vi "Do.vi"(8 "error in (no error)":errorcluster, 10 "Actor in":refnum<class "Actor.lvclass">, 11 "Configure Runt Trigger Source [RT] Msg":refnum<class "Configure Runt Trigger Source [RT] Msg.lvclass">) -> (0 "error out":errorcluster, 2 "Actor out":refnum<class "Actor.lvclass">)   [LabVIEW 2015, in "CS++Scope.lvlib" / "Configure Runt Trigger Source [RT] Msg.lvclass"]
doc: "This VI delivers the message to the actor by calling the appropriate method(s) on the actor."
uses:
  Configure Runt Trigger Source [RT] Msg.lvclass
  CS++Scope/CS++Scope.lvclass
  <vilib>/ActorFramework/Actor/Actor.lvclass
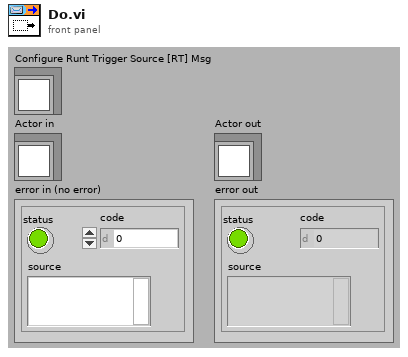
[diagram p1: front panel]
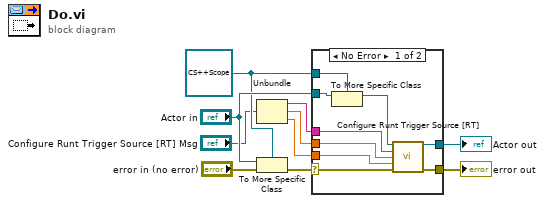
[diagram p0: block diagram]
diagram:
  w5 = refnum<class "CS++Scope.lvclass"> refnum ("Actor in")
  n1 = Unbundle ("Main-Unbundle")("Configure Runt Trigger Source [RT] Msg") -> (w3:string, w2:dbl[unit], w1:dbl[unit])
  n2 = To More Specific Class(target class=w5, reference="Actor in", error in="error in (no error)") -> (error out=w9:errorcluster)  [unwired: 1 out]
  n3 = case shown="No Error" w9 {
    selector: w9 -> [w17 w21]
    tunnel: [w19 w21] -> w8
    tunnel: [w18 w20] -> w7
    tunnel: "Actor in" -> [w16 w20]
    tunnel: w5 -> [w15 _]
    tunnel: w3 -> [w13 _]
    tunnel: w2 -> [w12 _]
    tunnel: w1 -> [w11 _]
    frame No Error {
      n4 = To More Specific Class(target class=w15, reference=w16) -> (specific class reference=w14:refnum<class "CS++Scope.lvclass">)  [unwired: 1 in, 1 out]
      n5 = call-dynamic "Configure Runt Trigger Source [RT].vi"("CS++Scope"=w14, "trigger source (\"CHANNEL1\")"=w13, "runt low threshold (1.0 V)"=w12, "runt high threshold (4.0 V)"=w11, "error in (no error)"=w17) -> ("CS++Scope out"=w18:refnum<class "CS++Scope.lvclass">, "error out"=w19:errorcluster)  [unwired: 9 in]
    }
    frame Error {
    }
  }
  "error out" <- w8
  "Actor out" <- w7
